vi "op_run.vi"(0 "Chain IN":bool, 1 "Dump Control":dbl, 5 "Left Drive":dbl, 7 "Right Drive":dbl, 9 "Arm Control":dbl, 11 "Lift String Control":dbl, 12 "Release Hang Lock":bool, 13 "Flag Raiser":bool, 14 "Flag Deployer":bool) -> (4 "Chain OUT":bool)   [LabVIEW 2010, in "LASA Beta.lvrbt"]
uses:
  LASA Beta.lvrbt
  <vilib>/NXT/NXTIO Xnodes/AddressXNode/NXTIOAddress.xnode
  <vilib>/NXT/Subs/MotorXNode.DC Motor Type.ctl
  <vilib>/NXT/Subs/MotorXNode.1DCMotor.ctl
  <vilib>/NXT/Subs/MotorXNode.Servo Type.ctl
  <vilib>/NXT/Subs/MotorXNode.1Servo.ctl
  <vilib>/NXT/Subs/MotorXNode.2Servo.ctl
  <vilib>/NXT/Subs/MotorXNode.2DCMotor.ctl
  <vilib>/NXT/Subs/LVHSConnector.ctl
  <vilib>/NXT/NXTIO Xnodes/NXTIOXNode/NXTIO.xnode
  <vilib>/NXT/NXTIO Xnodes/NXTIONodeSubVIs/TETRIX IO Move DC Motors.vi
  <vilib>/NXT/NXTIO Xnodes/NXTIONodeSubVIs/TETRIX IO Move Servos.vi
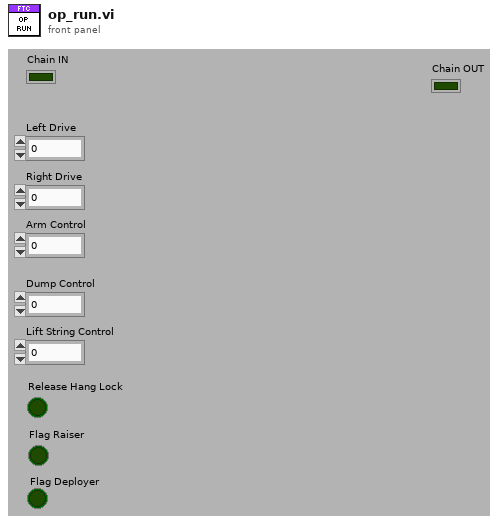
[diagram p1: front panel]
types:
  T1 = typedef "MotorXNode.DC Motor Type.ctl" = enum16{"DC Motor"}
  T2 = typedef "MotorXNode.Servo Type.ctl" = enum16{"Servo"}
  T3 = cluster{"Servo":T2, "Address":i16, "Address":i16}
  T4 = cluster{"DC Motor":T1, "Address":i16, "Address":i16}
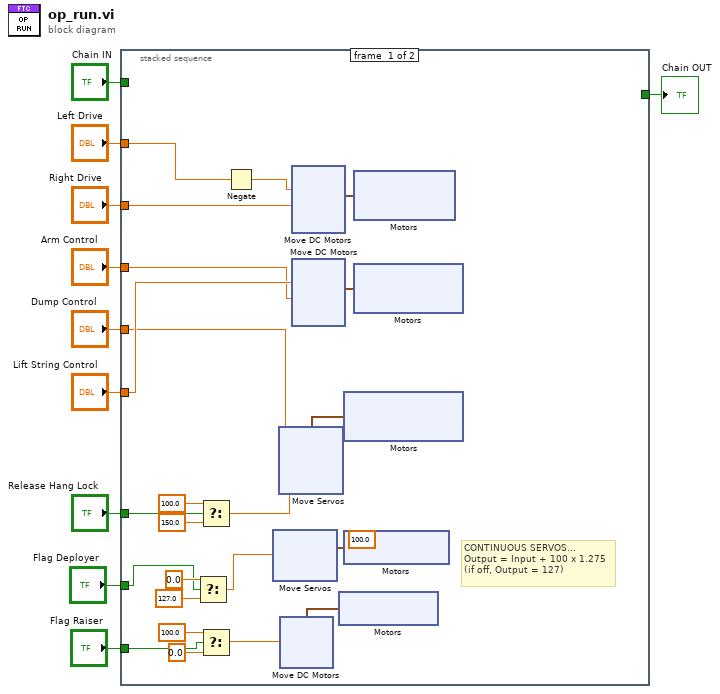
[diagram p0: block diagram]
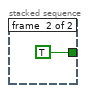
[diagram p2: hidden frame]
diagram:
  n1 = stacked-sequence {
    tunnel: "Left Drive" -> [w34 _]
    tunnel: "Right Drive" -> [w22 _]
    tunnel: "Arm Control" -> [w11 _]
    tunnel: "Dump Control" -> [w17 _]
    tunnel: "Lift String Control" -> [w20 _]
    tunnel: "Flag Deployer" -> [w25 _]
    tunnel: "Release Hang Lock" -> [w30 _]
    tunnel: "Flag Raiser" -> [w33 _]
    tunnel: [w28 _] -> _
    tunnel: "Chain IN" -> [w28 _]
    tunnel: [_ TRUE] -> w1
    frame #0 {
      (unwired) 100.0 ("t")
      # "CONTINUOUS SERVOS...\nOutput = Input + 100 x 1.275\n(if off, Output = 127)"
      n2 = Select(t=0.0, s=w25, f=127.0) -> (s? t:f=w15:dbl)
      n3 = Select(t=100.0, s=w30, f=150.0) -> (s? t:f=w16:dbl)
      n4 = Select(t=100.0, s=w33, f=0.0) -> (s? t:f=w19:dbl)
      n5 = Negate(x=w34) -> (-x=w23:dbl)
      n6 = xnode "Motors"() -> ("DC Motor"=w13:cluster{"DC Motor":T1, "Address":i16})
      n7 = xnode "Move DC Motors"("Power/Speed 1"=w19, "Motors"=w13) -> ()  [unwired: 1 in, 1 out]
      n8 = xnode "Motors"() -> ("Servo"=w18:T3)
      n9 = xnode "Move Servos"("Position 2"=w16, "Position 1"=w17, "Servos"=w18) -> ()  [unwired: 1 in, 1 out]
      n10 = xnode "Motors"() -> ("Servo"=w14:cluster{"Servo":T2, "Address":i16})
      n11 = xnode "Move Servos"("Position 1"=w15, "Servos"=w14) -> ()  [unwired: 1 in, 1 out]
      n12 = xnode "Motors"() -> ("DC Motor"=w24:T4)
      n13 = xnode "Move DC Motors"("Power/Speed 2"=w22, "Power/Speed 1"=w23, "Motors"=w24) -> ()  [unwired: 1 in, 1 out]
      n14 = xnode "Motors"() -> ("DC Motor"=w21:T4)
      n15 = xnode "Move DC Motors"("Power/Speed 2"=w11, "Power/Speed 1"=w20, "Motors"=w21) -> ()  [unwired: 1 in, 1 out]
    }
    frame #1 {
    }
  }
  "Chain OUT" <- w1
